vi "Shutdown.vi"(8 "error in":errorcluster, 11 "ePAS in":refnum<class "ePAS.lvclass">) -> (0 "error out":errorcluster, 3 "ePAS out":refnum<class "ePAS.lvclass">)   [LabVIEW 2014, in "ePAS Library.lvlib" / "ePAS.lvclass"]
doc: "General Instrument shutdown procedures. Kill open queues."
uses:
  ePAS.lvclass
  FPGA/Session/Exscalabar FPGA.lvclass
  ePAS.lvclass/ePAS.ctl
  reusable/PAS/Main/PAS.lvclass
  <userlib>/_Session Fwk/Session - Root.lvclass
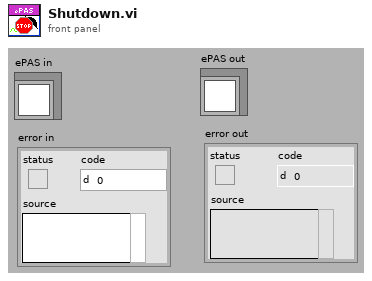
[diagram p1: front panel]
types:
  T1 = typedef "Session - Root.lvclass/Session Handle.ctl" = refnum<data-value>
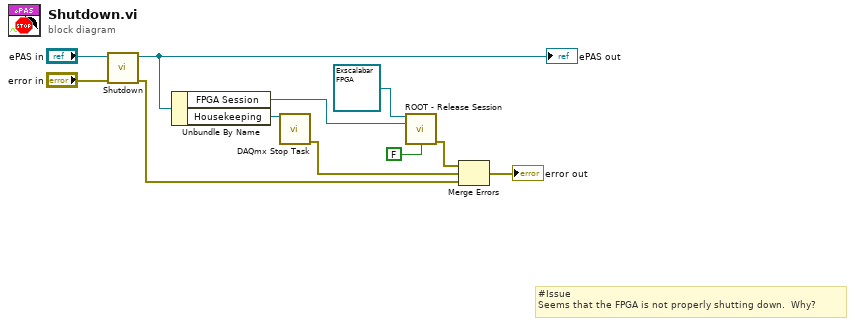
[diagram p0: block diagram]
diagram:
  # "#Issue\nSeems that the FPGA is not properly shutting down.  Why?"
  n1 = call-parent "Shutdown.vi"("error in"="error in", "Instrument in"="ePAS in") -> ("error out"=w5:errorcluster, "Instrument out"=w8:refnum<class "ePAS.lvclass">)  [unwired: 8 in]
  "ePAS out" <- w8
  n2 = Unbundle By Name(w8) -> ("FPGA Session"=w1:T1, "Housekeeping"=w9:refnum<k21>)
  n3 = call <vilib>:"DAQmx Stop Task.vi"("task/channels in"=w9) -> ("error out"=w4:errorcluster)  [unwired: 13 in, 1 out]
  n4 = call <userlib>:"ROOT - Release Session.vi"("OBJ - Session in"=refnum<class "Exscalabar FPGA.lvclass"> refnum ("Ex FPGA"), "Session Handle in"=w1, "force destroy? (F)"=FALSE) -> ("error out"=w3:errorcluster)  [unwired: 11 in, 1 out]
  n5 = Merge Errors(w3, w4, w5) -> (→"error out":errorcluster)
